vi "launcher-a.vi"() -> ()   [LabVIEW 2020]
uses:
  modules/reporting-device/reporting-device.lvlib
panel:
  in  "time-to-live":i32=100 caption="time-to-live-s"
  in  "period":i32=100 caption="period-ms"
  in  "show":bool
  in  "device-name":string[](array[string])=["cRIO-1", "cRIO-2", "cRIO-3"]
  in  "measurements":string[][](array[string])=[["temp1", "pressure1", "distance1"], ["temp2", "pressure2", "distance2"], ["temp3", "pressure3", "distance3"], ["temp4", "", "distance4"], ["temp5", "", "distance5"], ["temp6", "", ""]]
  in  "redis-server":cluster{"ip":string, "port":u16, "timeout":i32}={"ip"="localhost", "port"=6379, "timeout"=1000}
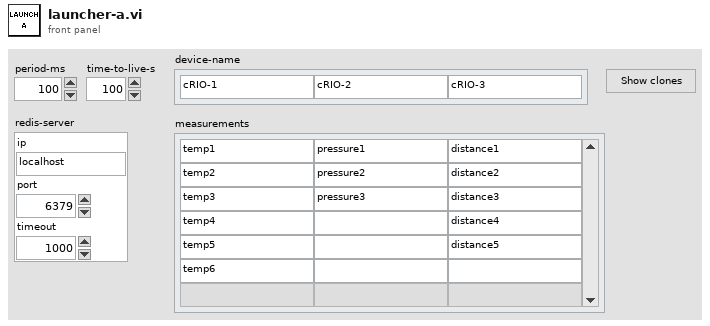
[diagram p1: front panel]
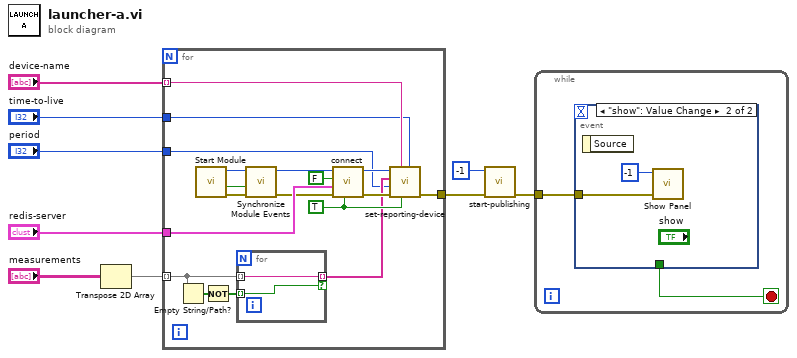
[diagram p0: block diagram]
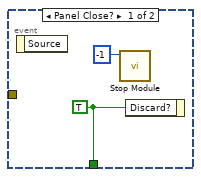
[diagram p2: hidden frame]
diagram:
  n1 = Transpose 2D Array(2D array="measurements") -> (transposed array=w7:string[][])
  n2 = for {
    tunnel: "redis-server" -> [w22]
    tunnel: w7 -> [w20] mode=indexing
    tunnel: [w12] -> w6
    tunnel: "device-name" -> [w13] mode=indexing
    tunnel: "period" -> [w11]
    tunnel: "time-to-live" -> [w10]
    w15 = TRUE ("wait for reply (T)")
    n3 = Empty String/Path?(string/path=w20) -> (empty?=w19:bool[])
    n4 = call "Start Module.vi"() -> ("error out"=w24:errorcluster, "Wait for Event Sync?"=w25:bool, "Module ID"=w26:i32)  [unwired: 8 in, 1 out]
    n5 = Not(x=w19) -> (.not. x?=w18:bool[])
    n6 = for {
      tunnel: w20 -> [w28] mode=indexing
      tunnel: [w28] -> w14 mode=indexing if=w27
      tunnel: w18 -> [w27] mode=indexing
    }
    n7 = call "Synchronize Module Events.vi"("error in"=w24, "Wait for Event Sync?"=w25, "Module ID in"=w26) -> ("error out"=w21:errorcluster, "Module ID out"=w17:i32)  [unwired: 7 in]
    n8 = call "connect.vi"("wait for reply (T)"=w15, "error in"=w21, "connection"=w22, "flush"=FALSE, "Module ID"=w17) -> ("error out"=w16:errorcluster)  [unwired: 4 in, 2 out]
    n9 = call "set-reporting-device.vi"("ttl"=w10, "wait for reply (T)"=w15, "device-name"=w13, "error in"=w16, "period-ms"=w11, "measurement-list"=w14, "Module ID"=w17) -> ("error out"=w12:errorcluster)  [unwired: 2 in, 2 out]
  }
  n10 = call "start-publishing.vi"("error in"=w6, "Module ID"=-1) -> ("error out"=w4:errorcluster)  [unwired: 6 in, 3 out]
  n11 = while {
    tunnel: w4 -> [w29]
    stop <- w30 stop-if-true
    n12 = event shown="[1] \"show\": Value Change" {
      selector: _ -> [_ _]
      dyn-events: _ -> [_ _]
      timeout: _ -> [_ _]
      tunnel: [w32 _] -> w30
      tunnel: w29 -> [_ w34]
      event Panel Close? {
        w32 = TRUE ("Discard?")
        n13 = event-data() -> ()  [unwired: 1 in, 1 out]
        n14 = call "Stop Module.vi"("Module ID"=-1) -> ()  [unwired: 10 in, 1 out]
        n15 = event-data("Discard?"=w32) -> ()  [unwired: 1 in, 1 out]
      }
      event "show": Value Change {
        n16 = event-data() -> ()  [unwired: 1 in, 1 out]
        n17 = call "Show Panel.vi"("error in"=w34, "Module ID"=-1) -> ()  [unwired: 9 in, 1 out]
      }
    }
  }
